vi "Check Engine Blocks.vi"(8 "error in (no error)":errorcluster, 10 "previous channel block":T1={"string offset"=0, "string data type"=enum."Bool", "engine data type"=enum."Bool", "name"="", "settings"=[], "units"="V"} {"string offset" format="%d bytes"}, 11 "channel block":T1={"string offset"=0, "string data type"=enum."Bool", "engine data type"=enum."Bool", "name"="", "settings"=[], "units"="V"} {"string offset" format="%d bytes"}) -> (0 "error out":errorcluster)   [LabVIEW 2017, in "DSF Core.lvlib"]
uses:
  DSF Core.lvlib
  Typedefs/DSF Engine Channel Configuration.ctl
  Typedefs/DSF Data Type.ctl
  Typedefs/DSF Settings Info.ctl
  Configuration Session.lvclass
  Channel Overlap.vi
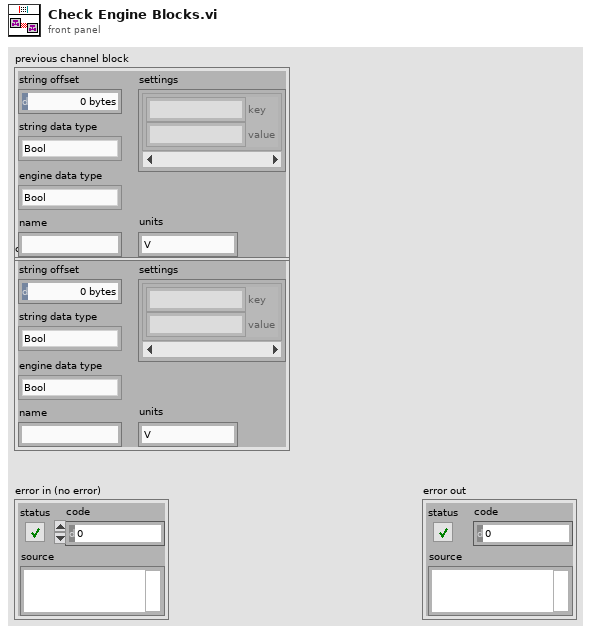
[diagram p1: front panel]
types:
  T1 = typedef "DSF Core.lvlib/DSF Engine Channel Configuration.ctl" = cluster{"string offset":u64, "string data type":T2, "engine data type":T2, "name":string, "settings":T3, "units":string}
  T2 = typedef "DSF Core.lvlib/DSF Data Type.ctl" = enum8{"Bool", "SGL", "DBL", "I8", "I16", "I32", "I64", "U8", "U16", "U32", "U64"}
  T3 = typedef "DSF Core.lvlib/DSF Settings Info.ctl" = cluster{"key":string, "value":string}[]
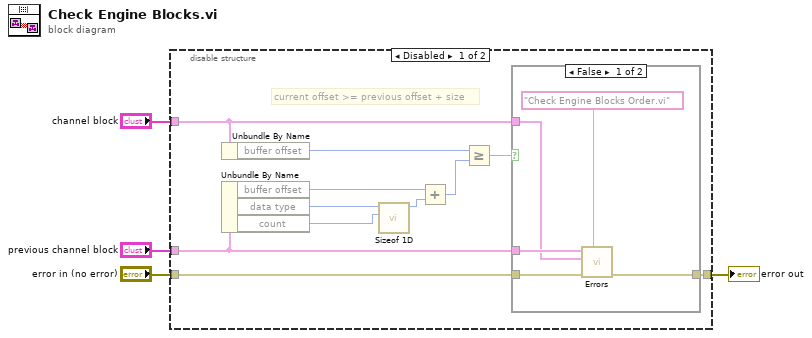
[diagram p0: block diagram]
diagram:
  n1 = disable-structure shown="Disabled" {
    disable-tunnel: "error in (no error)" -> [w15 _]
    disable-tunnel: [w14 _] -> w3
    disable-tunnel: "channel block" -> [w13 _]
    disable-tunnel: "previous channel block" -> [w9 _]
    frame Disabled {
      # "current offset >= previous offset + size"
      n2 = Unbundle By Name(w13) -> ("buffer offset"=w8:u64)
      n3 = Unbundle By Name(w9) -> ("buffer offset"=w11:u64, "data type"=w10:T2, "count"=w5:u64)
      n4 = call "Sizeof 1D.vi"("count"=w5, "data type"=w10) -> ("size in bytes"=w12:u64)  [unwired: 9 in]
      n5 = Add(x=w11, y=w12) -> (x+y=w7:u64)
      n6 = Greater Or Equal?(x=w8, y=w7) -> (x >= y?=w6:bool)
      n7 = case shown="False" w6 {
        tunnel: w9 -> [w20 _]
        tunnel: w13 -> [w19 _]
        tunnel: [w18 w21] -> w14
        tunnel: w15 -> [w17 w21]
        frame False {
          n8 = call-poly "Errors.vi"("error source vi name"="Check Engine Blocks Order.vi", "error in (no error)"=w17, "current channel block"=w19, "previous channel block"=w20) -> ("error out"=w18:errorcluster)  [unwired: 7 in]
        }
        frame True {
          # "Valid. Proceed."
        }
      }
    }
    frame Enabled {
    }
  }
  "error out" <- w3
